vi "DriveAutoTunePID_ReportRight.vi"(4 "Tuning in Progress":bool, 7 "Tuning Done in":bool, 8 "Diagnostic Info in":T1, 9 "Error Occured in":bool, 10 "Plant and Test Data in":T3, 11 "New Tuning Parameters in":T2) -> ()   [LabVIEW 2023]
uses:
  <vilib>/Rock Robotics/Network Tables/NT Get Topic.vi
  <vilib>/Rock Robotics/Network Tables/NT Get PublishHandle.vi
  <vilib>/Rock Robotics/Network Tables/NT_LL_Write Boolean.vi
  <vilib>/Rock Robotics/Network Tables/NT Check Errors.vi
  <vilib>/Rock Robotics/Network Tables/NT_LL_Write Number.vi
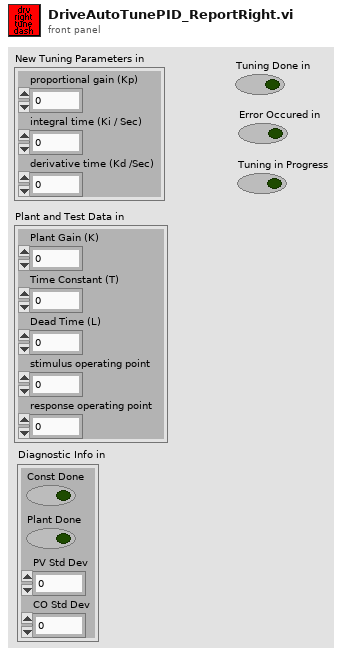
[diagram p1: front panel]
types:
  T1 = cluster{"Const Done":bool, "Plant Done":bool, "PV Std Dev":dbl, "CO Std Dev":dbl}
  T2 = cluster{"proportional gain (Kp)":dbl, "integral time (Ki / Sec)":dbl, "derivative time (Kd /Sec)":dbl}
  T3 = cluster{"Plant Gain (K)":dbl, "Time Constant (T)":dbl, "Dead Time (L)":dbl, "stimulus operating point":dbl, "response operating point":dbl}
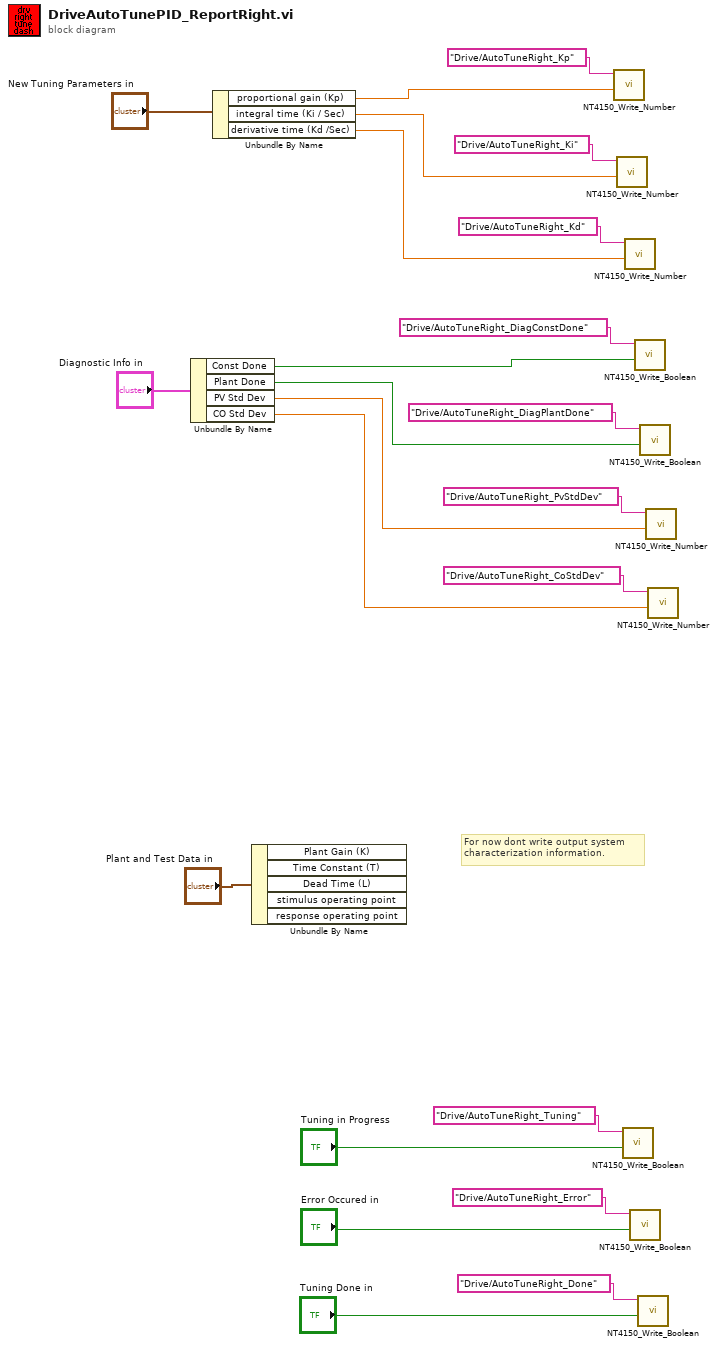
[diagram p0: block diagram]
diagram:
  # "For now dont write output system\ncharacterization information."
  n1 = Unbundle By Name("Diagnostic Info in") -> ("Const Done"=w7:bool, "Plant Done"=w6:bool, "PV Std Dev"=w5:dbl, "CO Std Dev"=w4:dbl)
  n2 = Unbundle By Name("New Tuning Parameters in") -> ("proportional gain (Kp)"=w14:dbl, "integral time (Ki / Sec)"=w13:dbl, "derivative time (Kd /Sec)"=w12:dbl)
  n3 = Unbundle By Name("Plant and Test Data in") -> ()  [unwired: 5 out]
  n4 = call "NT4150_Write_Number.vi"("value"=w14, "name"="Drive/AutoTuneRight_Kp") -> ()  [unwired: 9 in, 1 out]
  n5 = call "NT4150_Write_Number.vi"("value"=w13, "name"="Drive/AutoTuneRight_Ki") -> ()  [unwired: 9 in, 1 out]
  n6 = call "NT4150_Write_Boolean.vi"("value"="Tuning in Progress", "name"="Drive/AutoTuneRight_Tuning") -> ()  [unwired: 9 in, 1 out]
  n7 = call "NT4150_Write_Number.vi"("value"=w12, "name"="Drive/AutoTuneRight_Kd") -> ()  [unwired: 9 in, 1 out]
  n8 = call "NT4150_Write_Boolean.vi"("value"="Error Occured in", "name"="Drive/AutoTuneRight_Error") -> ()  [unwired: 9 in, 1 out]
  n9 = call "NT4150_Write_Boolean.vi"("value"=w7, "name"="Drive/AutoTuneRight_DiagConstDone") -> ()  [unwired: 9 in, 1 out]
  n10 = call "NT4150_Write_Boolean.vi"("value"="Tuning Done in", "name"="Drive/AutoTuneRight_Done") -> ()  [unwired: 9 in, 1 out]
  n11 = call "NT4150_Write_Boolean.vi"("value"=w6, "name"="Drive/AutoTuneRight_DiagPlantDone") -> ()  [unwired: 9 in, 1 out]
  n12 = call "NT4150_Write_Number.vi"("value"=w5, "name"="Drive/AutoTuneRight_PvStdDev") -> ()  [unwired: 9 in, 1 out]
  n13 = call "NT4150_Write_Number.vi"("value"=w4, "name"="Drive/AutoTuneRight_CoStdDev") -> ()  [unwired: 9 in, 1 out]
